vi "Fractional FFT.vi"(2 "alpha":cdb format="%.2f", 3 "X":cdb[](array[numeric]) format="%.2f") -> (0 "error":i32, 1 "Fract FFT {X}":cdb[](array[numeric]) format="%.2f")   [LabVIEW 2014, in "NI_Gmath.lvlib"]
doc: "Realizes the fractional fast Fourier transform of complex signals with arbitrarily chosen signal lengths.\n\nIt is\n\nFFFT{X}(j) = Sum exp(-2*pi*i*j*k*alpha)*xk\n\nwhere j and k run from 0 to length(X)."
uses:
  NI_Gmath.lvlib
  Complex FFT.vi
  Inverse Real FFT.vi
  NI_AALPro.lvlib
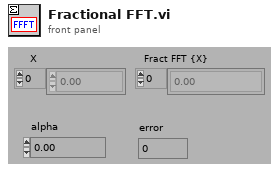
[diagram p1: front panel]
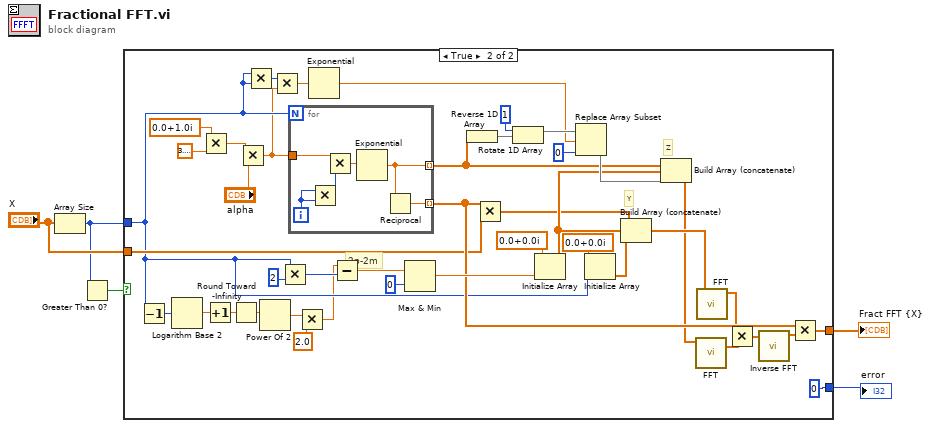
[diagram p0: block diagram]
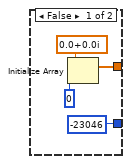
[diagram p2: hidden frame]
diagram:
  n1 = Array Size(array="X") -> (size(s)=w3:i32)
  n2 = Greater Than 0?(x=w3) -> (x > 0?=w2:bool)
  n3 = case shown="True" w2 {
    tunnel: [w6 w51] -> w4
    tunnel: "X" -> [_ w46]
    tunnel: w3 -> [_ w44]
    tunnel: [-23046 0] -> w1
    frame False {
      n4 = Initialize Array(cdb 0.0+0.0i, 0) -> (w6:cdb[])
    }
    frame True {
      # "2p-2m"
      # "Y"
      # "Z"
      n5 = Decrement(x=w44) -> (x-1=w45:i32)
      n6 = Logarithm Base 2(1:w45) -> (0:w14:dbl)
      n7 = Multiply(x=cdb 0.0+1.0i, y=3.141592653589793) -> (x*y=w19:cdb)
      n8 = Increment(x=w14) -> (x+1=w16:dbl)
      n9 = Round Toward -Infinity(1:w16) -> (0:w15:dbl)
      n10 = Multiply(x=w19, y="alpha") -> (x*y=w34:cdb)
      n11 = Multiply(x=w44, y=w44) -> (x*y=w33:i32)
      n12 = Power Of 2(x=w15) -> (2^x=w12:dbl)
      n13 = Multiply(x=w33, y=w34) -> (x*y=w35:cdb)
      n14 = Multiply(x=w44, y=2) -> (x*y=w23:i32)
      n15 = for {
        N: w44 -> [_]
        tunnel: w34 -> [w56]
        tunnel: [w53] -> w47 mode=indexing
        tunnel: [w52] -> w28 mode=indexing
        i -> [w57]
        n16 = Multiply(x=w57, y=w57) -> (x*y=w55:i32)
        n17 = Multiply(x=w56, y=w55) -> (x*y=w54:cdb)
        n18 = Exponential(1:w54) -> (0:w52:cdb)
        n19 = Reciprocal(x=w52) -> (1/x=w53:cdb)
      }
      n20 = Multiply(x=w12, y=2.0) -> (x*y=w22:dbl)
      n21 = Exponential(1:w35) -> (0:w10:cdb)
      n22 = Subtract(x=w22, y=w23) -> (x-y=w48:dbl)
      n23 = Max & Min(x=w48, y=0) -> (max(x,y)=w50:dbl)  [unwired: 1 out]
      n24 = Reverse 1D Array(array=w28) -> (reversed array=w29:cdb[])
      n25 = Multiply(x=w47, y=w46) -> (x*y=w25:cdb[])
      n26 = Rotate 1D Array(1:w29, 2:1) -> (0:w31:cdb[])
      n27 = Initialize Array(cdb 0.0+0.0i, w50) -> (w27:cdb[])
      n28 = Replace Array Subset(array=w31, new element=w10, index=0) -> (w36:cdb[])
      n29 = Initialize Array(cdb 0.0+0.0i, w44) -> (w26:cdb[])
      n30 = Build Array (concatenate)(w25, w27, w26) -> (w42:cdb[])
      n31 = Build Array (concatenate)(w28, w27, w36) -> (w41:cdb[])
      n32 = call-poly "FFT.vi"("X"=w41) -> ("FFT {X}"=w38:cdb[])  [unwired: 9 in, 1 out]
      n33 = call-poly "FFT.vi"("X"=w42) -> ("FFT {X}"=w37:cdb[])  [unwired: 9 in, 1 out]
      n34 = Multiply(x=w37, y=w38) -> (x*y=w39:cdb[])
      n35 = call-poly "Inverse FFT.vi"("FFT {X}"=w39) -> ("X"=w40:dbl[])  [unwired: 9 in, 1 out]
      n36 = Multiply(x=w47, y=w40) -> (x*y=w51:cdb[])
    }
  }
  "Fract FFT {X}" <- w4
  "error" <- w1
